vi "Separate Array Values.vi"() -> ()   [LabVIEW 2019]
doc: "This VI takes an input array that contains a mixture of positive and negative values and separates that array into two smaller arrays - one containing just the negative values and one containing just the positive values."
panel:
  out "Less than or Equal to Zero":dbl[](array[numeric])
  out "Greater than Zero":dbl[](array[numeric])
  in  "Input Array":dbl[](array[numeric])=[6.0, 3.9, -5.8, 0.0, -2.6, -1.0, 2.2, -4.3]
  # "Overview: Demonstrates iterating through elements of a one-dimensional array and building two output arrays, one of which contains all the elements above zero and one that contains all the elements less than or equal to zero.\nInstructions:\nRun the VI."
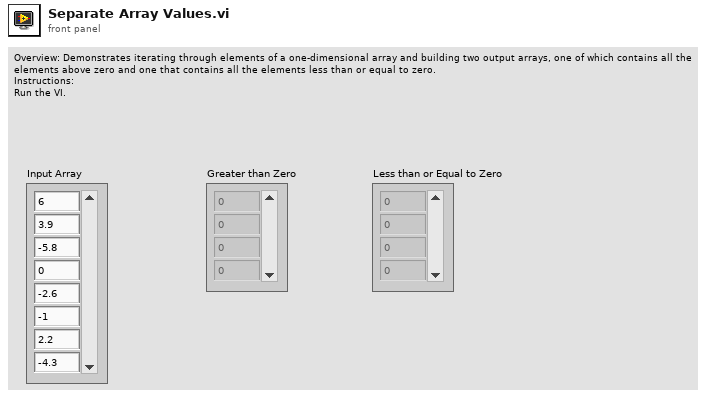
[diagram p1: front panel]
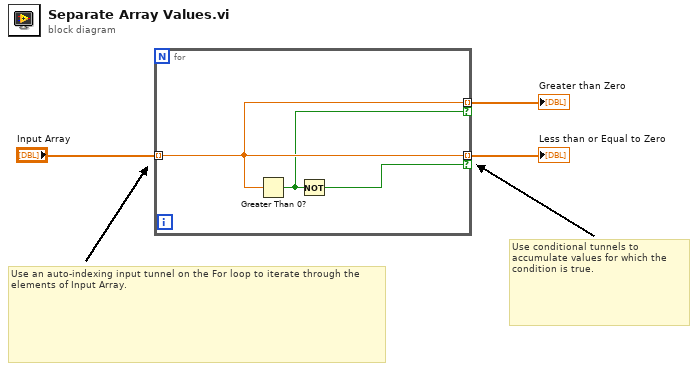
[diagram p0: block diagram]
diagram:
  # "Use conditional tunnels to accumulate values for which the condition is true."
  # "Use an auto-indexing input tunnel on the For loop to iterate through the elements of Input Array."
  n1 = for {
    tunnel: "Input Array" -> [w6] mode=indexing
    tunnel: [w6] -> w2 mode=indexing if=w5
    tunnel: [w6] -> w1 mode=indexing if=w4
    n2 = Greater Than 0?(x=w6) -> (x > 0?=w5:bool)
    n3 = Not(x=w5) -> (.not. x?=w4:bool)
  }
  "Greater than Zero" <- w2
  "Less than or Equal to Zero" <- w1
